vi "read typedef clusters for channel info.vi"() -> (0 "error out":errorcluster, 1 "Channel Counts":i32[](array[numeric]), 2 "> Categorized name list >":string[][](array[string]), 3 "> Uncategorized name list >":string[](array[string]))   [LabVIEW 2013, in "fixed channel tag bus module configuration.lvclass"]
uses:
  fixed channel tag bus module configuration.lvclass
  <vilib>/NI/Tag Bus Module Framework/channel/channel classification.ctl
  <vilib>/NI/Tag Bus Module Framework/channel/TBM channel.lvclass
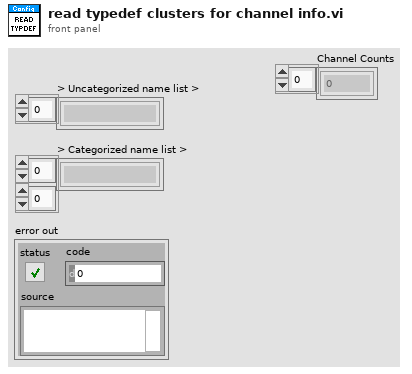
[diagram p1: front panel]
types:
  T1 = typedef "TBM channel.lvclass/channel classification.ctl" = enum16{"input data", "output data", "processing parameter", "processing result"}
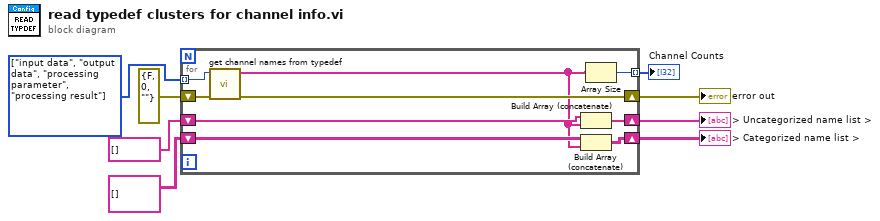
[diagram p0: block diagram]
diagram:
  w5 = T1[] [enum."input data", enum."output data", enum."processing parameter", enum."processing result"] items=["input data", "output data", "processing parameter", "processing result"]
  n1 = for {
    tunnel: w5 -> [w17] mode=indexing
    shift-right: [w16] -> w4
    shift-left: string[][] [] -> [w15]
    shift-right: [w14] -> w8
    shift-left: errorcluster {"status"=FALSE, "code"=0, "source"=""} ("error out") -> [w13]
    shift-right: [w12] -> w7
    shift-left: string[] [] -> [w11]
    tunnel: [w9] -> w1 mode=indexing
    n2 = call "get channel names from typedef.vi"("error in"=w13, "channel classification"=w17) -> ("error out"=w14:errorcluster, "Channel Names"=w10:string[])  [unwired: 8 in]
    n3 = Build Array (concatenate)(w11, w10) -> (w12:string[])
    n4 = Build Array (concatenate)(w15, w10) -> (w16:string[][])
    n5 = Array Size(array=w10) -> (size(s)=w9:i32)
  }
  "error out" <- w8
  "> Uncategorized name list >" <- w7
  "> Categorized name list >" <- w4
  "Channel Counts" <- w1
